vi "Fetch.vi"   [LabVIEW 2022 SP3, in "Keithley 2450.lvlib"]
doc: "Fetches acquired data from the instrument. The correct fetch subVI depends on the desired data."
uses:
  Keithley 2450.lvlib
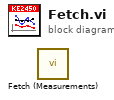
[diagram p0: block diagram]
diagram:
  n1 = call "Fetch (Measurements).vi"() -> ()  [unwired: 13 in, 3 out]
